vi "Test Skip Overrides Upstreams Fail Status.vi"(8 "error in (no error)":errorcluster, 11 "Test Assertion Results in":refnum<class "Assertion Result Test.lvclass">) -> (0 "error out":errorcluster, 3 "Test Assertion Results out":refnum<class "Assertion Result Test.lvclass">)   [LabVIEW 2020, in "LUnit Tests.lvlib" / "Assertion Result Test.lvclass"]
uses:
  Assertion Result Test.lvclass
  C:/Program Files (x86)/National Instruments/LabVIEW 2020/vi.lib/Asteme/LUnit/Test Case.lvclass
  Test Dummys/Test Case Test Double/Test Case Test Double.lvclass
  C:/Users/anton/Documents/GitHub/LUnit/source/Framework/Test Case/LUnit Test Case.lvclass
  source/Framework/Result Classes/Assertion Result/Public/TypeDefs/Status.ctl
  source/Framework/Test Case/LUnit Test Case.lvclass/LUnit Test Case.ctl
  source/Framework/Result Classes/Test Case Result/Test Case Result.lvclass/Test Case Result.ctl
  source/Framework/Result Classes/Method Result/Method Result.lvclass/Method Result.ctl
  <vilib>/Asteme/LUnit/Test Case.lvclass/Test Case.ctl
  <vilib>/Asteme/LUnit/LUnit Assertion Result.lvclass/LUnit Assertion Result.ctl
  <vilib>/Asteme/LUnit/LUnit Test Case Result.lvclass/LUnit Test Case Result.ctl
  <vilib>/Asteme/LUnit/LUnit Method Result.lvclass/LUnit Method Result.ctl
  source/Framework/Result Classes/Test Case Result/Private/SubVIs/Merge Status.vi
  <vilib>/Asteme/LUnit/Palette/Fail.vi
  <vilib>/Asteme/LUnit/Palette/Pass.vi
  <vilib>/Asteme/LUnit/Set Assertion Type.vi
  <vilib>/Asteme/LUnit/Add test result.vi
  <vilib>/Asteme/LUnit/LUnit Write Passed.vi
  <vilib>/Asteme/LUnit/LUnit Write Message.vi
  <vilib>/Asteme/LUnit/LUnit Write Description.vi
  <vilib>/Asteme/LUnit/LUnit Write Assertion Type.vi
  <vilib>/Asteme/LUnit/LUnit Record Assertion Result.vi
  <vilib>/Asteme/LUnit/LUnit Aggregate Assertion Results.vi
  <vilib>/Asteme/LUnit/Assertion Result/LUnit Read Status.vi
  <vilib>/Asteme/LUnit/LUnit Read Message.vi
  <vilib>/Asteme/LUnit/LUnit Read Description.vi
  <vilib>/Asteme/LUnit/Method Result/LUnit Merge Status.vi
  <vilib>/Asteme/LUnit/LUnit Concatenate result strings.vi
  <vilib>/Asteme/LUnit/LUnit Assertion Result.lvclass
  source/Framework/Test Case/LUnit Test Case.lvclass
  source/Framework/Result Classes/Test Case Result/Test Case Result.lvclass
  <vilib>/Asteme/LUnit/Test Case.lvclass
  source/Framework/Result Classes/Assertion Result/Assertion Result.lvclass
  C:/Users/anton/Documents/GitHub/LUnit/tests/Test Dummys/Test Case Test Double/Test Case Test Double.lvclass
  C:/Users/anton/Documents/GitHub/LUnit/tests/Framework Test/Test Assertion Results/Assertion Result Test.lvclass
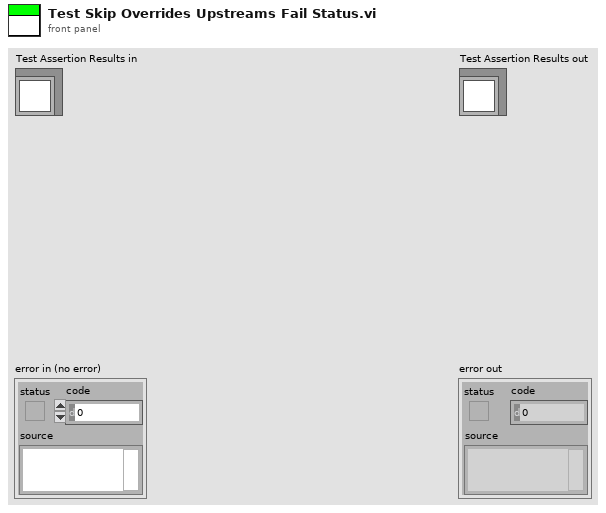
[diagram p1: front panel]
types:
  T1 = typedef "Assertion Result.lvclass/Status.ctl" = enum16{"Pass", "Fail", "Error", "Skipped", "Setup Error", "Broken", "Teardown Error"}
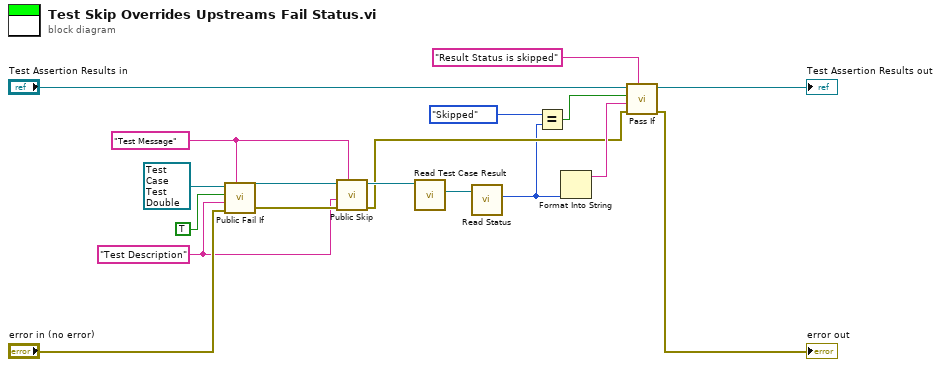
[diagram p0: block diagram]
diagram:
  w11 = "Test Message" ("Description")
  w12 = "Test Description" ("Description")
  n1 = call "Public Fail If.vi"("Message"=w11, "error in (no error)"="error in (no error)", "Description"=w12, "Fail?"=TRUE, "Test Case Test Double in"=refnum<class "Test Case Test Double.lvclass"> refnum ("Test Case Test Double.lvclass")) -> ("error out"=w14:errorcluster, "Test Case Test Double out"=w13:refnum<class "Test Case Test Double.lvclass">)  [unwired: 5 in]
  n2 = call "Public Skip.vi"("Description"=w11, "error in (no error)"=w14, "Message"=w12, "Test Case Test Double in"=w13) -> ("error out"=w5:errorcluster, "Test Case Test Double out"=w10:refnum<class "Test Case Test Double.lvclass">)  [unwired: 6 in]
  n3 = call "Read Test Case Result.vi"("LUnit Test Case In"=w10) -> ("Test Case Result"=w9:refnum<class "Test Case Result.lvclass">)  [unwired: 9 in, 1 out]
  n4 = call "Read Status.vi"("Test Case Result In"=w9) -> ("Status"=w3:T1)  [unwired: 8 in, 2 out]
  n5 = Equal?(x=Status."Skipped" ("y"), y=w3) -> (x = y?=w1:bool)
  n6 = Format Into String(w3) -> (resulting string=w6:string)  [unwired: 3 in, 1 out]
  n7 = call <vilib>:"Pass If.vi"("Description"="Result Status is skipped", "error in (no error)"=w5, "Message"=w6, "Pass?"=w1, "LUnit Test Case In"="Test Assertion Results in") -> ("error out"=→"error out":errorcluster, "LUnit Test Case Out"=→"Test Assertion Results out":refnum<class "Assertion Result Test.lvclass">)  [unwired: 5 in]
